vi "Watchdog Occurance.vi"() -> ()   [LabVIEW 2015]
doc: "This RT VI uses an FPGA personality to control a watchdog timer. One loop runs every Wait (ms) to kick the watchdog. The Timeout (ms) regulates how often the watchdog needs to be kicked in order to avoid a watchdog expiration.\n\nIf the watchdog isn't kicked within the timeout period specified while the Arm control is set, an interrupt is set. This interrupt triggers a dialog to indicate that the watchdog has expired. This dialog can be replaced with code for a more real-world application, such as resetting a hardware device upon watchdog expiration."
uses:
  <vilib>/FPGAPlugInAG/sbRIO-9637/niLvFpga_Open_sbRIO-9637.vi
  <vilib>/Utility/error.llb/Error Cluster From Error Code.vi
  <vilib>/RVI Host/nirviSupport.llb/nirviErrorClusterFromErrorCode.vi
  <vilib>/rvi/errors/niLvFpgaAdjustHostInterfaceError.vi
  <vilib>/FPGAPlugInAG/sbRIO-9637/niLvFpga_Close_sbRIO-9637.vi
  <vilib>/rvi/interface/nirviOpenFPGA/nirviOpenFPGA.xnode
  FPGA Bitfiles/WDOccurance-sbRI_FPGATarget_WDPolling_gzBYnV6Png8.lvbitx
  <vilib>/rvi/interface/nirviMethod/nirviMethod.xnode
  <vilib>/rvi/interface/nirviReadWriteControl/nirviReadWriteControl.xnode
  <vilib>/rvi/interface/nirviCloseFPGA/nirviCloseFPGA.xnode
  NiFpgaLv.dll
  <vilib>/FPGAPlugInAG/sbRIO-9637/niLvFpga_AcknowledgeIrq_sbRIO-9637.vi
  <vilib>/rvi/interface/nirviMethod/StockFPGA_InlinedMethodWaitForSingleIRQ.vi
  <vilib>/FPGAPlugInAG/sbRIO-9637/niLvFpga_WaitOnIrq_sbRIO-9637.vi
panel:
  out "Number of whacks":i32
  in  "Stop":bool
  in  "Arm":bool
  in  "Timeout (ms)":u32=100
  in  "Wait (ms)":u32=50
  # "This RT VI uses an FPGA personality to control a watchdog timer. A watchdog\nloop runs every Wait (ms) to whack the watchdog. The Timeout (ms) \nregulates how often the watchdog needs to be whacked in order to avoid\na watchdog expiration.\nIf the watchdog isn't whacked within the timeout period specified while\nthe Arm control is set, an interrupt is sent from the FPGA to RT. This interrupt \ntriggers a dialog to indicate that the watchdog has expired. This dialog can \nbe replaced with code in a real-world application, such as resetting a \nhardware device upon watchdog expiration. To stop the VI, press the stop\nbutton and after 10 seconds of inactivity, the interrupt will timeout and end."
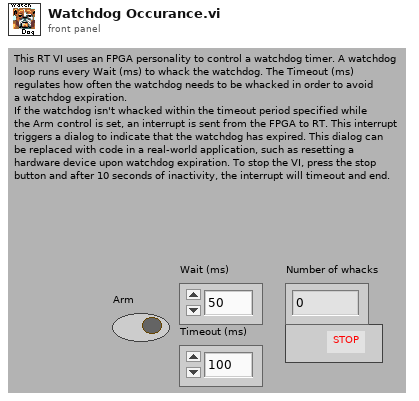
[diagram p1: front panel]
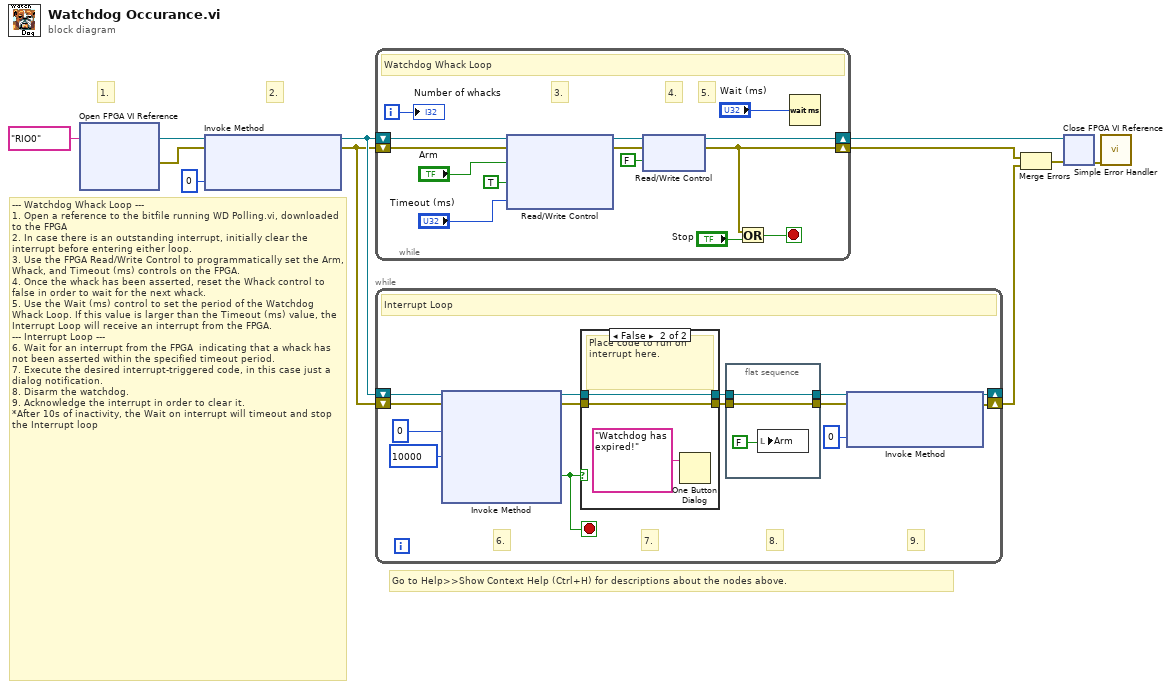
[diagram p0: block diagram]
diagram:
  # "2."
  # "1."
  # "Go to Help>>Show Context Help (Ctrl+H) for descriptions about the nodes above."
  # "--- Watchdog Whack Loop ---\n1. Open a reference to the bitfile running WD Polling.vi, downloaded to the FPGA\n2. In case there is an outstanding interrupt, initially clear the interrupt before entering either loop.\n3. Use the FPGA Read/Write Control to programmatically set the Arm, Whack, and Timeout (ms) controls on the FPGA.\n4. Once the whack has been asserted, reset the Whack control to false in order to wait for the next whack.\n5. Use the Wait (ms) control to set the period of the Watchdog Whack Loop. If this value is larger than the Timeout (ms) value, the Interrupt Loop will receive an interrupt from the FPGA.\n--- Interrupt Loop ---\n6. Wait for an interrupt from the FPGA  indicating that a whack has not been asserted within the specified timeout period.\n7. Execute the desired interrupt-triggered code, in this case just a dialog notification.\n8. Disarm the watchdog.\n9. Acknowledge the interrupt in order to clear it.\n*After 10s of inactivity, the Wait on interrupt will timeout and stop the Interrupt loop"
  n1 = xnode "Open FPGA VI Reference"("resource name"=tag "RIO0") -> ("FPGA VI Reference Out"=w2:refnum<k20>, "error out"=w1:errorcluster)  [unwired: 1 in]
  n2 = xnode "Invoke Method"("FPGA VI Reference In"=w2, "error in"=w1, "IRQ Number(s)"=0) -> ("FPGA VI Reference Out"=w10:refnum<k20>, "error out"=w9:errorcluster)
  n3 = while {
    shift-right: [w12] -> w5
    shift-left: w9 -> [w24]
    shift-right: [w16] -> w11
    shift-left: w10 -> [w25]
    i -> [w13]
    stop <- w18 stop-if-true
    # "5."
    # "4."
    # "3."
    # "Watchdog Whack Loop"
    n4 = xnode "Read/Write Control"("FPGA VI Reference In"=w25, "error in"=w24, "Arm"="Arm", "Whack"=TRUE, "Timeout (ms)"="Timeout (ms)") -> ("FPGA VI Reference Out"=w15:refnum<k20>, "error out"=w14:errorcluster)
    n5 = xnode "Read/Write Control"("FPGA VI Reference In"=w15, "error in"=w14, "Whack"=FALSE) -> ("FPGA VI Reference Out"=w16:refnum<k20>, "error out"=w12:errorcluster)
    n6 = Or(x=w12, y="Stop") -> (x .or. y?=w18:bool)
    n7 = Wait (ms)(milliseconds to wait="Wait (ms)") -> ()  [unwired: 1 out]
    "Number of whacks" <- w13
  }
  n8 = while {
    shift-right: [w27] -> _
    shift-left: w10 -> [w37]
    shift-right: [w26] -> w4
    shift-left: w9 -> [w36]
    stop <- w32 stop-if-true
    # "9."
    # "8."
    # "7."
    # "6."
    # "Interrupt Loop"
    n9 = xnode "Invoke Method"("FPGA VI Reference In"=w37, "error in"=w36, "IRQ Number(s)"=0, "Timeout (ms)"=10000) -> ("FPGA VI Reference Out"=w34:refnum<k20>, "error out"=w33:errorcluster, "Timed Out"=w32:bool)  [unwired: 1 out]
    n10 = case shown="False" w32 {
      tunnel: [w44 w46] -> w31
      tunnel: [w43 w45] -> w29
      tunnel: w33 -> [w43 w45]
      tunnel: w34 -> [w44 w46]
      frame True {
      }
      frame False {
        # "Place code to run on interrupt here."
        n11 = One Button Dialog(message="Watchdog has expired!") -> ()  [unwired: 2 out]
      }
    }
    n12 = flat-sequence {
      tunnel: w31 -> [w41]
      tunnel: [w41] -> w30
      tunnel: w29 -> [w40]
      tunnel: [w40] -> w28
      frame #0 {
        n13 = local write "Arm"(FALSE) -> ()
      }
    }
    n14 = xnode "Invoke Method"("FPGA VI Reference In"=w30, "error in"=w28, "IRQ Number(s)"=0) -> ("FPGA VI Reference Out"=w27:refnum<k20>, "error out"=w26:errorcluster)
  }
  n15 = Merge Errors(w5, w4) -> (w6:errorcluster)
  n16 = xnode "Close FPGA VI Reference"("FPGA VI Reference In"=w11, "error in"=w6) -> ("error out"=w7:errorcluster)
  n17 = call <vilib>:"Simple Error Handler.vi"("error in (no error)"=w7) -> ()  [unwired: 4 in, 5 out]
